vi "Agilent VNA Calibrate.vi"(7 "Agilent VNA":T5, 8 "error in (no error)":errorcluster, 10 "Parameters to Measure":T1[](array[typedef]) {"Channel" min=1 max=99 step=1; "Parameter"."Stimulus Port" min=1 step=1; "Parameter"."Response Port" min=1 step=1}, 11 "VISA Resource Name":refnum<visa-resource-name>) -> (0 "error out":errorcluster {"code" format="%.0x"}, 3 "dup VISA Resource Name":refnum<visa-resource-name>)   [LabVIEW 2011]
uses:
  TypeDefs/Agilent VNA Instrument Info.ctl
  tests/S Parameter/TypeDefs/SP Parameter to Measure.ctl
  tests/S Parameter/TypeDefs/SP Parameter.ctl
  tests/S Parameter/TypeDefs/SP Calibration State.ctl
  tests/S Parameter/TypeDefs/SP Measurement Format.ctl
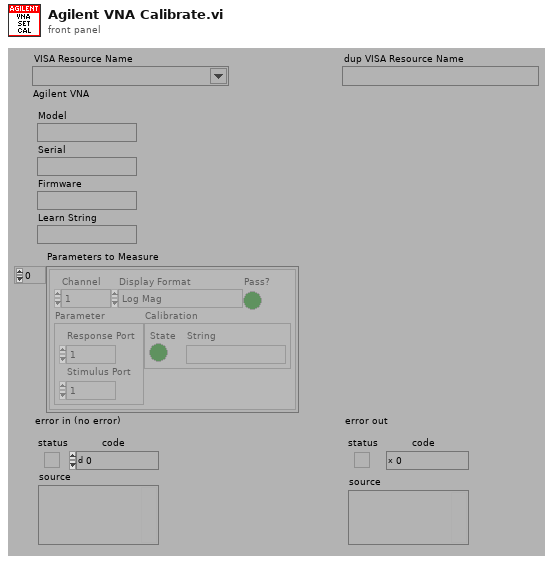
[diagram p1: front panel]
types:
  T1 = typedef "SP Parameter to Measure.ctl" = cluster{"Channel":i8, "Parameter":T2, "Calibration":T3, "Display Format":T4, "Pass?":bool}
  T2 = typedef "SP Parameter.ctl" = cluster{"Stimulus Port":i8, "Response Port":i8}
  T3 = typedef "SP Calibration State.ctl" = cluster{"State":bool, "String":string}
  T4 = typedef "SP Measurement Format.ctl" = enum32{"Log Mag", "Phase", "Delay", "Smith (R+jX)", "Polar (Re/Im)", "Linear Mag", "SWR", "Real", "Imaginary", "Smith (Lin/Phase)", "Smith (Log/Phase)", "Smith (Real/Imag)", "Smith (G+jB)", "Polar (Lin/Phase)", "Polar (Log/Phase)", "Expanded Phase", "Positive Phase", "Inverted Smith", "Unwrapped Phase", "Power Out", "Power In", "Linear Mag/Phase", "Log Mag/Phase", "Real/Imaginary"}
  T5 = typedef "Agilent VNA Instrument Info.ctl" = cluster{"Model":string, "Serial":string, "Firmware":string, "Learn String":string}
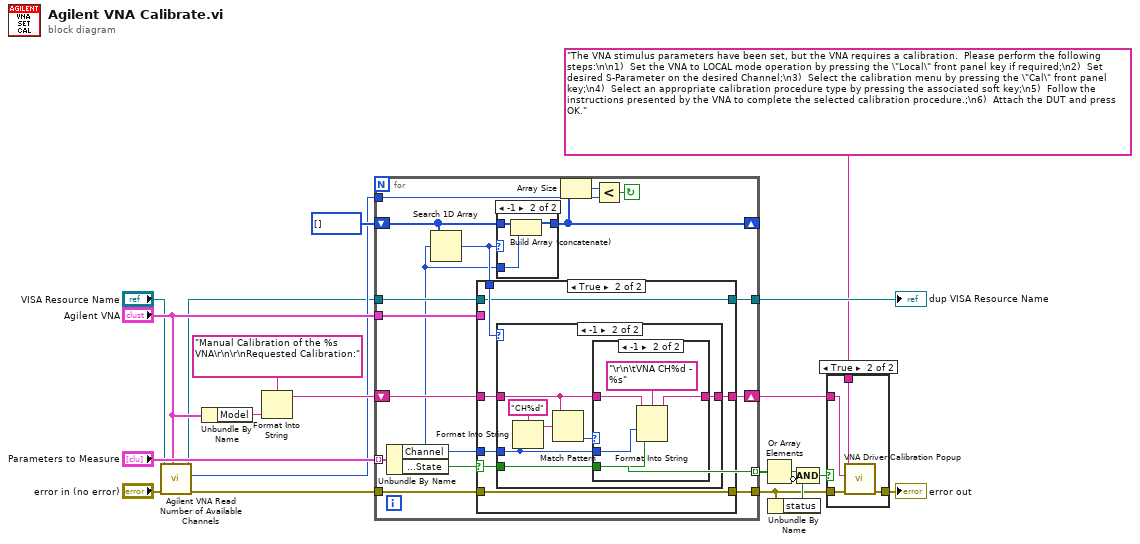
[diagram p0: block diagram]
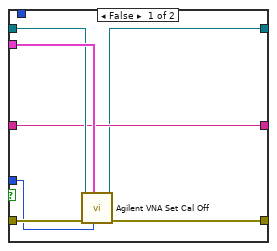
[diagram p3: hidden frame]
diagram:
  n1 = call "Agilent VNA Read Number of Available Channels.vi"("Agilent VNA"="Agilent VNA", "error in (no error)"="error in (no error)", "VISA Resource Name"="VISA Resource Name") -> ("error out"=w9:errorcluster, "Number of Channels"=w8:i8, "dup VISA Resource Name"=w6:refnum<visa-resource-name>)  [unwired: 6 out]
  n2 = Unbundle By Name("Agilent VNA") -> ("Model"=w17:string)
  n3 = Format Into String(format string="Manual Calibration of the %s VNA\r\n\r\nRequested Calibration:", w17) -> (resulting string=w18:string)  [unwired: 2 in, 1 out]
  n4 = for {
    shift-right: [w35] -> w12
    shift-left: w18 -> [w36]
    tunnel: "Parameters to Measure" -> [w34] mode=indexing
    tunnel: "Agilent VNA" -> [w32]
    tunnel: w6 -> [w33]
    tunnel: w9 -> [w31]
    tunnel: [w30] -> w1
    shift-right: [w28] -> _
    shift-left: i8[] [] -> [w29]
    tunnel: w8 -> [w26]
    tunnel: [w24] -> w15
    tunnel: [w22] -> w5 mode=indexing
    stop <- w21 continue-if-true
    n5 = Unbundle By Name(w34) -> ("Channel"=w23:i8, "Calibration.State"=w22:bool)
    n6 = Search 1D Array(1D array=w29, element=w23) -> (index of element=w25:i32)  [unwired: 1 out]
    n7 = case shown="True" w22 {
      selector: w22 -> [_ w51]
      tunnel: w36 -> [w43 w52]
      tunnel: [w43 w54] -> w35
      tunnel: w23 -> [w41 w50]
      tunnel: w33 -> [w46 w48]
      tunnel: w32 -> [w47 _]
      tunnel: w31 -> [w45 w53]
      tunnel: [w44 w53] -> w30
      tunnel: w25 -> [_ w49]
      tunnel: [w42 w48] -> w24
      frame False {
        n8 = call "Agilent VNA Set Cal Off.vi"("Channel"=w41, "Agilent VNA"=w47, "error in (no error)"=w45, "VISA Resource Name"=w46) -> ("error out"=w44:errorcluster, "dup VISA Resource Name"=w42:refnum<visa-resource-name>)  [unwired: 6 out]
      }
      frame True {
        n9 = case shown="-1" w49 {
          tunnel: [w55 w62] -> w54
          tunnel: w52 -> [w55 w61]
          tunnel: w51 -> [_ w60]
          tunnel: w50 -> [_ w58]
          frame Default {
          }
          frame -1 {
            n10 = Format Into String(format string="CH%d", w58) -> (resulting string=w59:string)  [unwired: 2 in, 1 out]
            n11 = Match Pattern(string=w61, regular expression=w59) -> (offset past match=w56:i32)  [unwired: 4 out]
            n12 = case shown="-1" w56 {
              tunnel: [w63 w67] -> w62
              tunnel: w61 -> [w63 w66]
              tunnel: w60 -> [_ w65]
              tunnel: w58 -> [_ w64]
              frame Default {
              }
              frame -1 {
                n13 = Format Into String(format string="\r\n\tVNA CH%d - %s", initial string=w66, w64, w65) -> (resulting string=w67:string)  [unwired: 1 in, 1 out]
              }
            }
          }
        }
      }
    }
    n14 = case shown="-1" w25 {
      tunnel: w29 -> [w37 w40]
      tunnel: [w37 w39] -> w28
      tunnel: w23 -> [_ w38]
      frame Default {
      }
      frame -1 {
        n15 = Build Array (concatenate)(w40, w38) -> (w39:i8[])
      }
    }
    n16 = Array Size(array=w28) -> (size(s)=w27:i32)
    n17 = Less?(x=w27, y=w26) -> (x < y?=w21:bool)
  }
  "dup VISA Resource Name" <- w15
  n18 = Or Array Elements(Boolean array=w5) -> (logical OR=w4:bool)
  n19 = Unbundle By Name(w1) -> ("status"=w3:bool)
  n20 = Compound Arithmetic op=AND(w4, invert w3) -> (w2:bool)
  n21 = case shown="True" w2 {
    tunnel: "The VNA stimulus parameters have been set, but the VNA requires a calibration.  Please perform the following steps:\n\n1)  Set the VNA to LOCAL mode operation by pressing the \"Local\" front panel key if required;\n2)  Set desired S-Parameter on the desired Channel;\n3)  Select the calibration menu by pressing the \"Cal\" front panel key;\n4)  Select an appropriate calibration procedure type by pressing the associated soft key;\n5)  Follow the instructions presented by the VNA to complete the selected calibration procedure.;\n6)  Attach the DUT and press OK." -> [_ w72]
    tunnel: [w69 w73] -> w20
    tunnel: w12 -> [_ w71]
    tunnel: w1 -> [w69 w70]
    frame False {
    }
    frame True {
      n22 = call "VNA Driver Calibration Popup.vi"("error in (no error)"=w70, "RequestedCal"=w71, "Message (\"\")"=w72) -> ("error out"=w73:errorcluster)  [unwired: 8 out]
    }
  }
  "error out" <- w20
